vi "Generate code.vi"(1 "Terms":T1[](array[typedef]), 3 "Diagram":refnum<vi>, 5 "XRef":refnum<vi>, 6 "State In":T4) -> (0 "Generated Code?":bool, 2 "State Out":T4, 4 "Reply":string[](array[string]))   [LabVIEW 2012, in "IsA.xnode"]
uses:
  IsA.xnode
  State.ctl
  <vilib>/XNodeSupport/XNodeTermIDPair.ctl
  <vilib>/XNodeSupport/XNodeTermRef.ctl
  <vilib>/XNodeSupport/XNodeString.ctl
  Scripting Tools.lvlib
  <vilib>/XNodeSupport/NI_XNodeSupport.lvlib
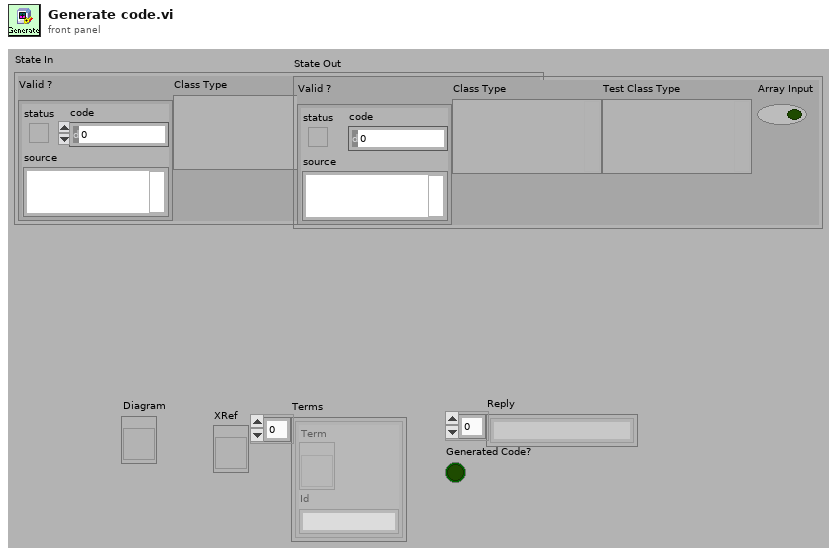
[diagram p1: front panel]
types:
  T1 = typedef "NI_XNodeSupport.lvlib/XNodeTermIDPair.ctl" = cluster{"Term":T2, "Id":T3}
  T2 = typedef "NI_XNodeSupport.lvlib/XNodeTermRef.ctl" = refnum<vi>
  T3 = typedef "NI_XNodeSupport.lvlib/XNodeString.ctl" = string
  T4 = typedef "IsA.xnode/State.ctl" = cluster{"Valid ?":errorcluster, "Class Type":variant, "Test Class Type":variant, "Array Input":bool}
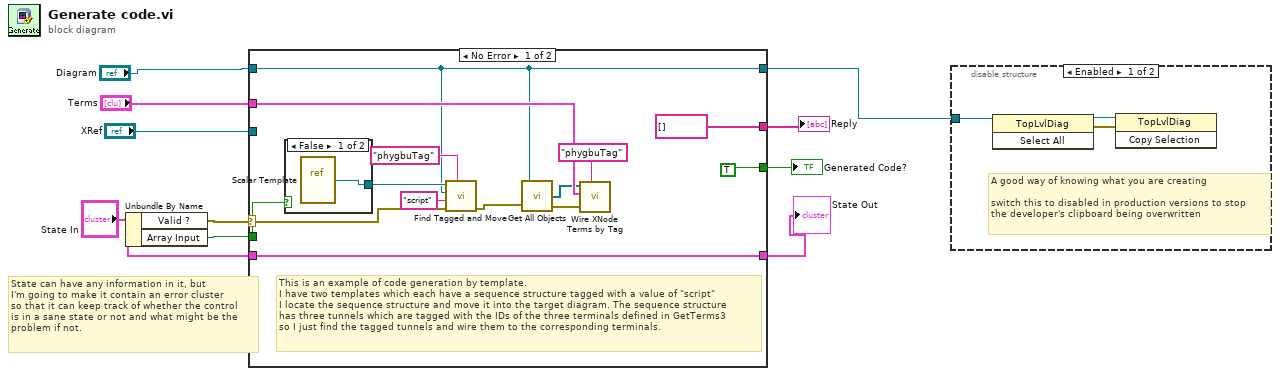
[diagram p0: block diagram]
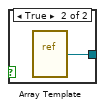
[diagram p2: hidden frame]
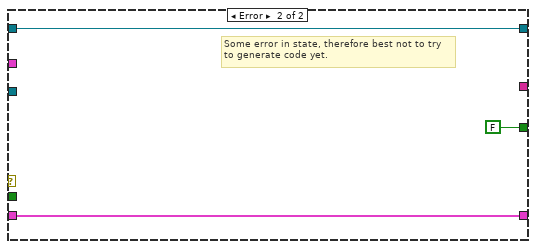
[diagram p3: hidden frame]
diagram:
  # "State can have any information in it, but\nI'm going to make it contain an error cluster\nso that it can keep track of whether the control\nis in a sane state or not and what might be the\nproblem if not."
  n1 = Unbundle By Name("State In") -> ("Valid ?"=w10:errorcluster, "Array Input"=w1:bool)
  n2 = case shown="No Error" w10 {
    selector: w10 -> [w19 _]
    tunnel: "State In" -> [w22 w29]
    tunnel: "Diagram" -> [w12 w27]
    tunnel: "Terms" -> [w16 _]
    tunnel: "XRef" -> [_ _]
    tunnel: [w12 w27] -> w2
    tunnel: [string[] [] ("Reply") _] -> w5
    tunnel: [TRUE FALSE] -> w4
    tunnel: [w22 w29] -> w3
    tunnel: w1 -> [w21 _]
    frame No Error {
      # "This is an example of code generation by template.\nI have two templates which each have a sequence structure tagged with a value of \"script\"\nI locate the sequence structure and move it into the target diagram. The sequence structure\nhas three tunnels which are tagged with the IDs of the three terminals defined in GetTerms3\nso I just find the tagged tunnels and wire them to the corresponding terminals."
      n3 = case shown="False" w21 {
        tunnel: [w25 w26] -> w20
        frame False {
          n4 = vi-ref "Scalar Template.vi"() -> (w25:refnum<vi>)
        }
        frame True {
          n5 = vi-ref "Array Template.vi"() -> (w26:refnum<vi>)
        }
      }
      n6 = call "Find Tagged and Move.vi"("TagName"="phygbuTag", "error in"=w19, "TagValue"="script", "Destination Diagram"=w12, "VI Refnum"=w20) -> ("error out"=w14:errorcluster)  [unwired: 1 in, 5 out]
      n7 = call "Get All Objects.vi"("Diagram In"=w12, "error in"=w14) -> ("All Objects"=w11:refnum<vi>[], "error out"=w13:errorcluster)  [unwired: 1 out]
      n8 = call "Wire XNode Terms by Tag.vi"("TagName"="phygbuTag", "error in (no error)"=w13, "Term Refs"=w16, "Source References"=w11) -> ()  [unwired: 8 out]
    }
    frame Error {
      # "Some error in state, therefore best not to try\nto generate code yet."
    }
  }
  "State Out" <- w3
  "Reply" <- w5
  "Generated Code?" <- w4
  n9 = disable-structure shown="Enabled" {
    disable-tunnel: w2 -> [w30 _]
    frame Enabled {
      # "A good way of knowing what you are creating\n\nswitch this to disabled in production versions to stop\nthe developer's clipboard being overwritten"
      n10 = invoke class="TopLvlDiag" method="Select All"(reference=w30) -> (reference out=w32:refnum<vi>, error out=w31:errorcluster)  [unwired: 2 in, 1 out]
      n11 = invoke class="TopLvlDiag" method="Copy Selection"(reference=w32, error in=w31) -> ()  [unwired: 1 in, 3 out]
    }
    frame Disabled {
    }
  }
